vi "ParamReader2.vi"(8 "error in (no error)":errorcluster, 10 "what kind of binary":i32, 11 "selected path":path caption="selected \"*.par\" path") -> (0 "error out":errorcluster, 2 "CodeString":string, 5 "Cluster":T1 {"AdcOffset" format="%#.6f"; "AdcScale" format="%#.6f"})   [LabVIEW 2014]
panel:
  out "slow ADC\nactiveChannels\nRange":string
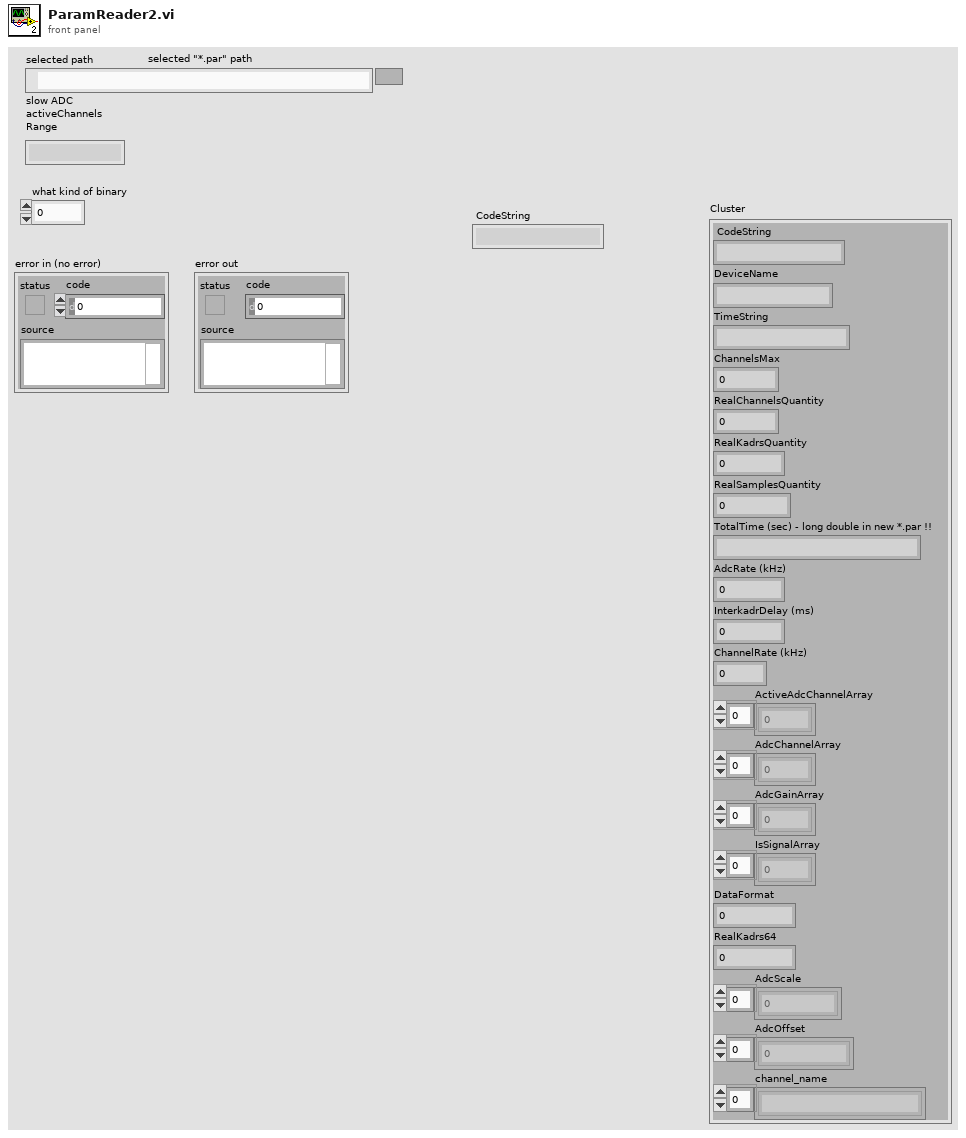
[diagram p1: front panel]
types:
  T1 = cluster{" CodeString":string, "DeviceName":string, "TimeString":string, "ChannelsMax":i16, "RealChannelsQuantity":i16, "RealKadrsQuantity":i64, "RealSamplesQuantity":i64, "TotalTime (sec) - long double in new *.par !!":string, "AdcRate (kHz)":dbl, "InterkadrDelay (ms)":dbl, "ChannelRate (kHz)":dbl, "ActiveAdcChannelArray":u32[], "AdcChannelArray":u8[], "AdcGainArray":u8[], "IsSignalArray":u8[], "DataFormat":i32, "RealKadrs64":i64, "AdcScale":dbl[], "AdcOffset":dbl[], "channel_name":string[]}
  T2 = enum16{"open", "replace", "create", "open or create", "replace or create", "replace or create with confirmation"}
  T3 = enum16{"deny read/write", "deny write-only", "deny none"}
  T4 = enum16{"big-endian, network order", "native, host order", "little-endian"}
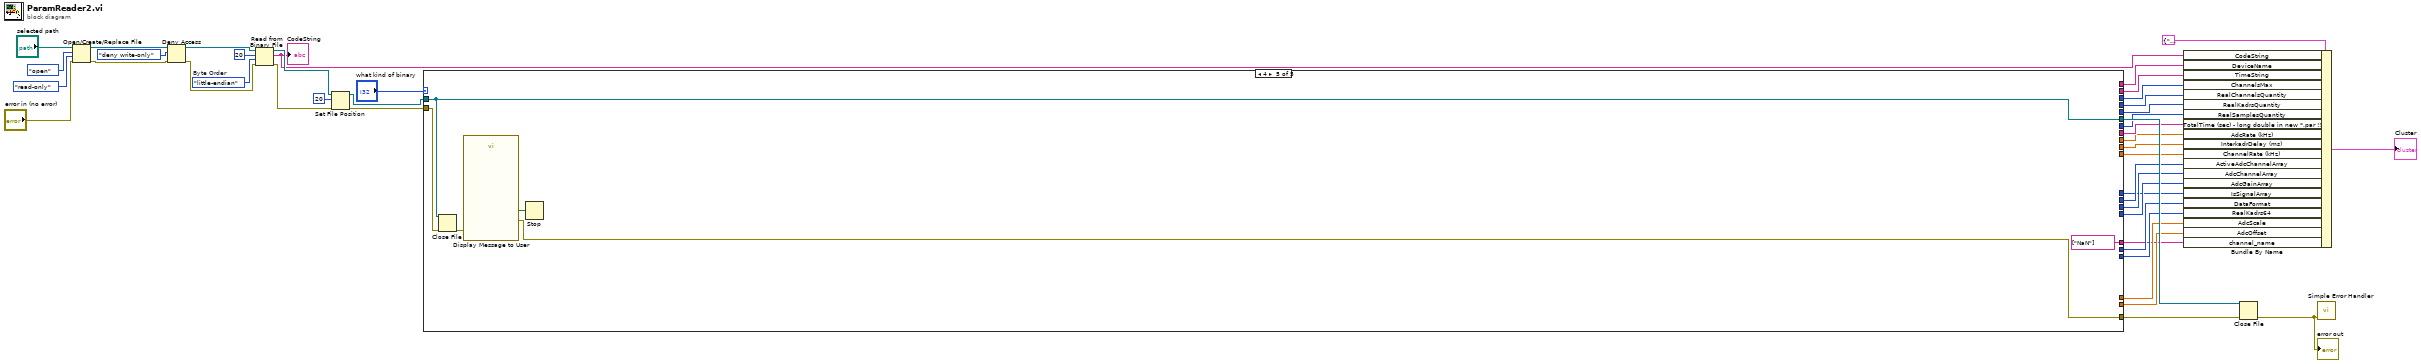
[diagram p0: block diagram]
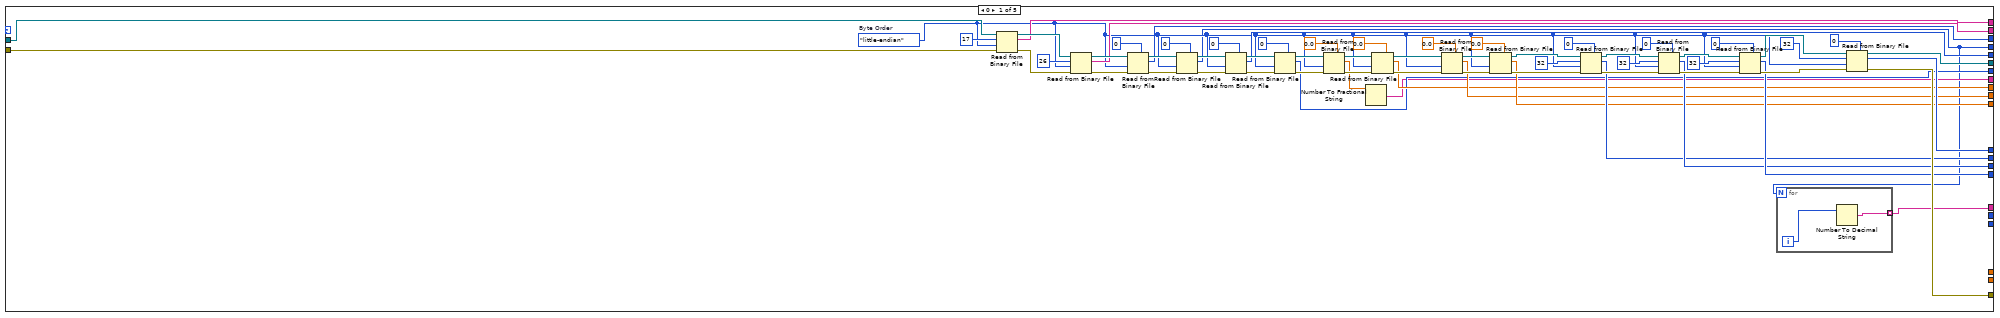
[diagram p2: hidden frame]
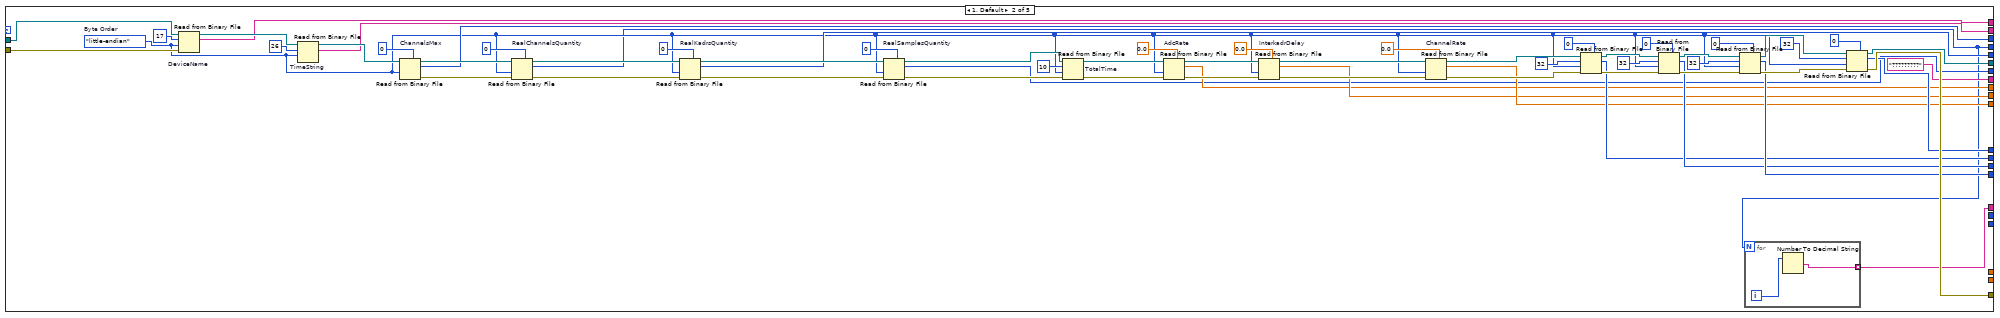
[diagram p3: hidden frame]
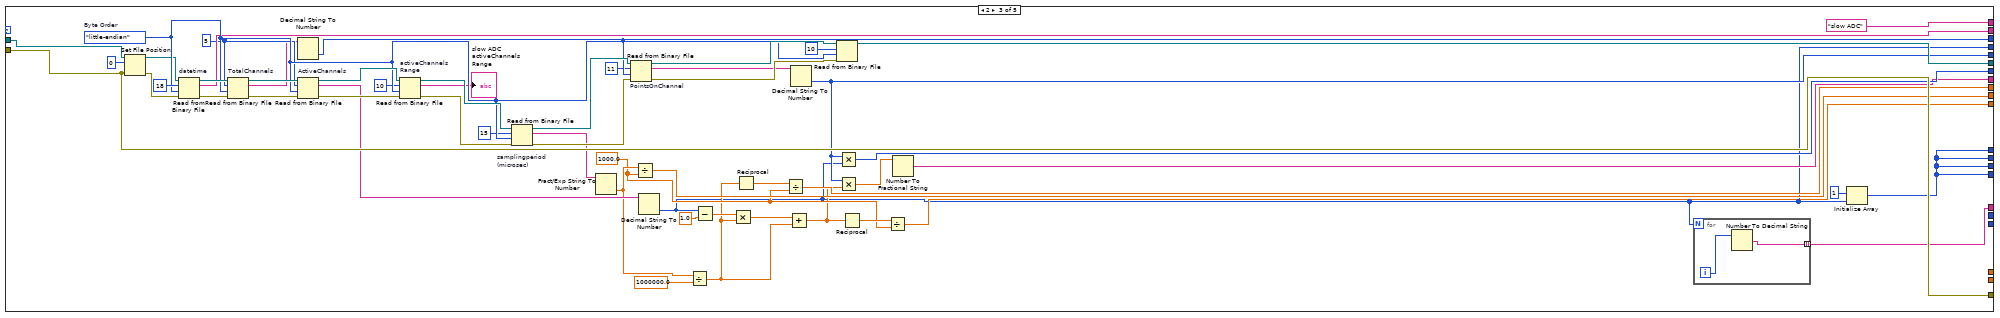
[diagram p4: hidden frame]
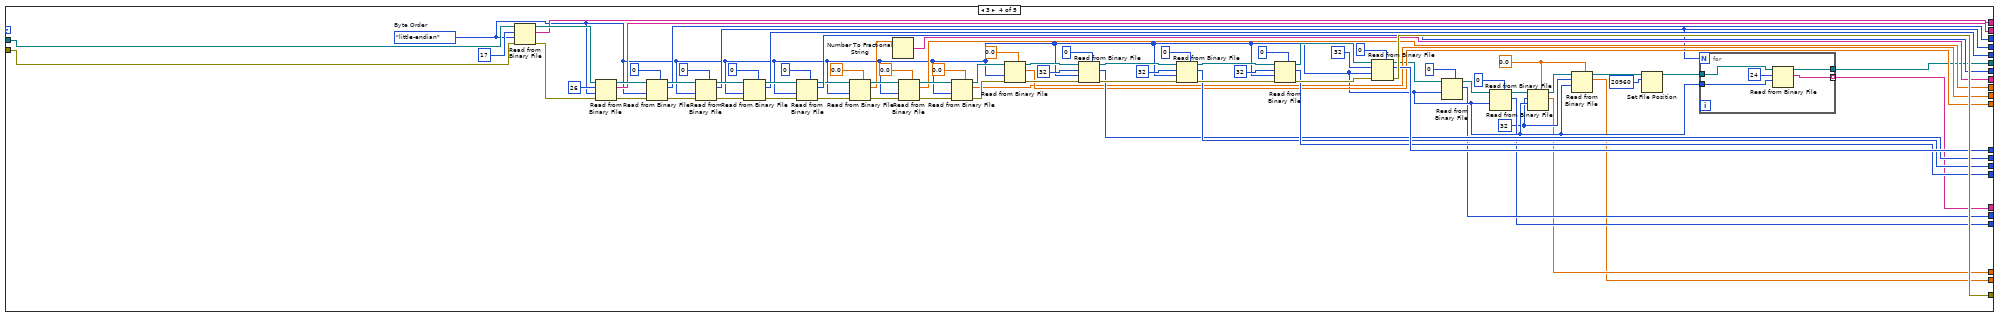
[diagram p5: hidden frame]
diagram:
  w29 = T4."little-endian"  # Byte Order
  n1 = Open/Create/Replace File(file path (use dialog)="selected path", error in="error in (no error)", operation (0:open)=T2."open", access (0:read/write)=enum16{"read/write", "read-only", "write-only"}."read-only") -> (refnum out=w31:refnum<file>, error out=w30:errorcluster)  [unwired: 2 in, 1 out]
  n2 = Deny Access(4:w30, 6:T3."deny write-only" ("deny mode (0:deny read/write)"), 7:w31) -> (0:w35:errorcluster, 3:w34:refnum<file>)
  n3 = Read from Binary File(8:w35, 9:w29, 10:20 ("count (1)"), 11:w34) -> (0:w39:errorcluster, 2:w20:string, 3:w37:refnum<file>)  [unwired: 2 in, 1 out]
  "CodeString" <- w20
  n4 = Set File Position(offset (in bytes) (0)=i64 20, refnum=w37, error in=w39) -> (refnum out=w41:refnum<file>, error out=w40:errorcluster)  [unwired: 1 in]
  n5 = case shown="4" "what kind of binary" {
    tunnel: w41 -> [w107 w171 w212 w309 w316]
    tunnel: [w66 w127 w208 w268 w318] -> w36
    tunnel: w40 -> [w106 w170 w208 w308 w320]
    tunnel: [w65 w126 w205 w248 w316] -> w42
    tunnel: [w64 w125 w185 w267 _] -> w6
    tunnel: [w63 w124 w185 w266 _] -> w7
    tunnel: [w62 w123 w185 w265 _] -> w8
    tunnel: [w61 w122 w185 w264 _] -> w9
    tunnel: [w60 w121 w181 w263 _] -> w10
    tunnel: [w59 w120 w189 w262 _] -> w11
    tunnel: [w58 w119 w191 w261 _] -> w12
    tunnel: [w57 w118 w190 w260 _] -> w14
    tunnel: [w56 w117 w177 w259 _] -> w15
    tunnel: [w44 w110 w174 w246 _] -> w16
    tunnel: [w55 w116 w198 w247 _] -> w17
    tunnel: [w54 w115 w207 w258 _] -> w18
    tunnel: [w53 w114 "slow ADC" w257 _] -> w19
    tunnel: [w49 "?????????" w178 w253 _] -> w13
    tunnel: [w43 w111 w175 w245 string[] ["NaN"]] -> w1
    tunnel: [_ _ _ w235 _] -> w5
    tunnel: [_ _ _ w234 _] -> w4
    tunnel: [_ _ _ w231 _] -> w3
    tunnel: [_ _ _ w230 _] -> w2
    frame 0 {
      w45 = T4."little-endian"  # Byte Order
      n6 = Read from Binary File(8:w106, 9:w45, 10:17 ("count (1)"), 11:w107) -> (0:w46:errorcluster, 2:w53:string, 3:w103:refnum<file>)  [unwired: 2 in, 1 out]
      n7 = Read from Binary File(8:w46, 9:w45, 10:26 ("count (1)"), 11:w103) -> (0:w47:errorcluster, 2:w54:string, 3:w101:refnum<file>)  [unwired: 2 in, 1 out]
      n8 = Read from Binary File(5:i16 0 ("count (1)"), 8:w47, 9:w45, 11:w101) -> (0:w88:errorcluster, 2:w55:i16, 3:w99:refnum<file>)  [unwired: 2 in, 1 out]
      n9 = Read from Binary File(5:i16 0 ("count (1)"), 8:w88, 9:w45, 11:w99) -> (0:w93:errorcluster, 2:w44:i16, 3:w92:refnum<file>)  [unwired: 2 in, 1 out]
      n10 = Read from Binary File(5:0 ("count (1)"), 8:w93, 9:w45, 11:w92) -> (0:w90:errorcluster, 2:w56:i32, 3:w91:refnum<file>)  [unwired: 2 in, 1 out]
      n11 = Read from Binary File(5:0 ("count (1)"), 8:w90, 9:w45, 11:w91) -> (0:w89:errorcluster, 2:w57:i32, 3:w51:refnum<file>)  [unwired: 2 in, 1 out]
      n12 = Read from Binary File(5:0.0 ("count (1)"), 8:w89, 9:w45, 11:w51) -> (0:w85:errorcluster, 2:w48:dbl, 3:w50:refnum<file>)  [unwired: 2 in, 1 out]
      n13 = Number To Fractional String(number=w48) -> (F-format string=w49:string)  [unwired: 3 in]
      n14 = Read from Binary File(5:sgl 0.0 ("count (1)"), 8:w85, 9:w45, 11:w50) -> (0:w84:errorcluster, 2:w58:sgl, 3:w87:refnum<file>)  [unwired: 2 in, 1 out]
      n15 = Read from Binary File(5:sgl 0.0 ("count (1)"), 8:w84, 9:w45, 11:w87) -> (0:w83:errorcluster, 2:w59:sgl, 3:w86:refnum<file>)  [unwired: 2 in, 1 out]
      n16 = Read from Binary File(5:sgl 0.0 ("count (1)"), 8:w83, 9:w45, 11:w86) -> (0:w79:errorcluster, 2:w60:sgl, 3:w80:refnum<file>)  [unwired: 2 in, 1 out]
      n17 = Read from Binary File(5:u8 0 ("count (1)"), 8:w79, 9:w45, 10:32 ("count (1)"), 11:w80) -> (0:w69:errorcluster, 2:w61:u8[], 3:w72:refnum<file>)  [unwired: 1 in, 1 out]
      n18 = Read from Binary File(5:u8 0 ("count (1)"), 8:w69, 9:w45, 10:32 ("count (1)"), 11:w72) -> (0:w68:errorcluster, 2:w62:u8[], 3:w71:refnum<file>)  [unwired: 1 in, 1 out]
      n19 = Read from Binary File(5:u8 0 ("count (1)"), 8:w68, 9:w45, 10:32 ("count (1)"), 11:w71) -> (0:w67:errorcluster, 2:w63:u8[], 3:w70:refnum<file>)  [unwired: 1 in, 1 out]
      n20 = for {
        N: w44 -> [_]
        tunnel: [w109] -> w43 mode=indexing
        i -> [w108]
        n21 = Number To Decimal String(number=w108) -> (decimal integer string=w109:string)  [unwired: 1 in]
      }
      n22 = Read from Binary File(5:u8 0 ("count (1)"), 8:w67, 9:w45, 10:32 ("count (1)"), 11:w70) -> (0:w66:errorcluster, 2:w64:u8[], 3:w65:refnum<file>)  [unwired: 1 in, 1 out]
    }
    frame 1, Default {
      w112 = T4."little-endian"  # Byte Order
      n23 = Read from Binary File "DeviceName"(8:w170, 9:w112, 10:17 ("count (1)"), 11:w171) -> (2:w114:string, 3:w167:refnum<file>)  [unwired: 2 in, 2 out]
      n24 = Read from Binary File "TimeString"(9:w112, 10:26 ("count (1)"), 11:w167) -> (2:w115:string, 3:w165:refnum<file>)  [unwired: 3 in, 2 out]
      n25 = Read from Binary File "ChannelsMax"(5:i16 0 ("count (1)"), 9:w112, 11:w165) -> (0:w150:errorcluster, 2:w116:i16, 3:w163:refnum<file>)  [unwired: 3 in, 1 out]
      n26 = Read from Binary File "RealChannelsQuantity"(5:i16 0 ("count (1)"), 8:w150, 9:w112, 11:w163) -> (0:w156:errorcluster, 2:w110:i16, 3:w155:refnum<file>)  [unwired: 2 in, 1 out]
      n27 = Read from Binary File "RealKadrsQuantity"(5:i64 0 ("count (1)"), 8:w156, 9:w112, 11:w155) -> (0:w152:errorcluster, 2:w117:i64, 3:w154:refnum<file>)  [unwired: 2 in, 1 out]
      n28 = Read from Binary File "RealSamplesQuantity"(5:i64 0 ("count (1)"), 8:w152, 9:w112, 11:w154) -> (0:w151:errorcluster, 2:w118:i64, 3:w153:refnum<file>)  [unwired: 2 in, 1 out]
      n29 = Read from Binary File "TotalTime"(8:w151, 9:w112, 10:10 ("count (1)"), 11:w153) -> (0:w146:errorcluster, 3:w149:refnum<file>)  [unwired: 2 in, 2 out]
      n30 = Read from Binary File "AdcRate"(5:0.0 ("count (1)"), 8:w146, 9:w112, 11:w149) -> (0:w145:errorcluster, 2:w119:dbl, 3:w148:refnum<file>)  [unwired: 2 in, 1 out]
      n31 = Read from Binary File "InterkadrDelay"(5:0.0 ("count (1)"), 8:w145, 9:w112, 11:w148) -> (0:w144:errorcluster, 2:w120:dbl, 3:w147:refnum<file>)  [unwired: 2 in, 1 out]
      n32 = Read from Binary File "ChannelRate"(5:0.0 ("count (1)"), 8:w144, 9:w112, 11:w147) -> (0:w140:errorcluster, 2:w121:dbl, 3:w141:refnum<file>)  [unwired: 2 in, 1 out]
      n33 = Read from Binary File(5:u32 0 ("count (1)"), 8:w140, 9:w112, 10:32 ("count (1)"), 11:w141) -> (0:w130:errorcluster, 2:w122:u32[], 3:w133:refnum<file>)  [unwired: 1 in, 1 out]
      n34 = Read from Binary File(5:u8 0 ("count (1)"), 8:w130, 9:w112, 10:32 ("count (1)"), 11:w133) -> (0:w129:errorcluster, 2:w123:u8[], 3:w132:refnum<file>)  [unwired: 1 in, 1 out]
      n35 = Read from Binary File(5:u8 0 ("count (1)"), 8:w129, 9:w112, 10:32 ("count (1)"), 11:w132) -> (0:w128:errorcluster, 2:w124:u8[], 3:w131:refnum<file>)  [unwired: 1 in, 1 out]
      n36 = for {
        N: w110 -> [_]
        tunnel: [w173] -> w111 mode=indexing
        i -> [w172]
        n37 = Number To Decimal String(number=w172) -> (decimal integer string=w173:string)  [unwired: 1 in]
      }
      n38 = Read from Binary File(5:u8 0 ("count (1)"), 8:w128, 9:w112, 10:32 ("count (1)"), 11:w131) -> (0:w127:errorcluster, 2:w125:u8[], 3:w126:refnum<file>)  [unwired: 1 in, 1 out]
    }
    frame 2 {
      w187 = 1000.0 ("y")
      w204 = 5 ("count (1)")
      w215 = T4."little-endian"  # Byte Order
      n39 = Set File Position(offset (in bytes) (0)=i64 0, refnum=w212, error in=w208) -> (refnum out=w210:refnum<file>, error out=w209:errorcluster)  [unwired: 1 in]
      n40 = Read from Binary File "datetime"(8:w209, 9:w215, 10:18 ("count (1)"), 11:w210) -> (0:w214:errorcluster, 2:w207:string, 3:w226:refnum<file>)  [unwired: 2 in, 1 out]
      n41 = Read from Binary File "TotalChannels"(8:w214, 9:w215, 10:w204, 11:w226) -> (0:w213:errorcluster, 2:w200:string, 3:w225:refnum<file>)  [unwired: 2 in, 1 out]
      n42 = Decimal String To Number(string=w200) -> (number=w198:i32)  [unwired: 2 in, 1 out]
      n43 = Read from Binary File "ActiveChannels"(8:w213, 9:w215, 10:w204, 11:w225) -> (0:w216:errorcluster, 2:w199:string, 3:w224:refnum<file>)  [unwired: 2 in, 1 out]
      n44 = Read from Binary File "activeChannels\nRange"(8:w216, 9:w215, 10:10 ("count (1)"), 11:w224) -> (0:w222:errorcluster, 2:→"slow ADC\nactiveChannels\nRange":string, 3:w221:refnum<file>)  [unwired: 2 in, 1 out]
      n45 = Read from Binary File "samplingperiod\n(microsec)"(8:w222, 9:w215, 10:i64 15 ("count (1)"), 11:w221) -> (0:w218:errorcluster, 2:w195:string, 3:w220:refnum<file>)  [unwired: 2 in, 1 out]
      n46 = Fract/Exp String To Number(string=w195) -> (number=w188:dbl)  [unwired: 3 in, 1 out]
      n47 = Read from Binary File "PointsOnChannel"(8:w218, 9:w215, 10:i64 11 ("count (1)"), 11:w220) -> (0:w217:errorcluster, 2:w197:string, 3:w219:refnum<file>)  [unwired: 2 in, 1 out]
      n48 = Divide(x=w188, y=w187) -> (x/y=w189:dbl)
      n49 = Decimal String To Number(string=w199) -> (number=w174:i32)  [unwired: 2 in, 1 out]
      n50 = Divide(x=w188, y=1000000.0) -> (x/y=w180:dbl)
      n51 = Subtract(x=w174, y=1.0) -> (x-y=w183:dbl)
      n52 = Multiply(x=w183, y=w180) -> (x*y=w182:dbl)
      n53 = Reciprocal(x=w180) -> (1/x=w192:dbl)
      n54 = Divide(x=w192, y=w187) -> (x/y=w191:dbl)
      n55 = Add(x=w182, y=w180) -> (x+y=w176:dbl)
      n56 = Decimal String To Number(string=w197) -> (number=w177:i32)  [unwired: 2 in, 1 out]
      n57 = Read from Binary File(8:w217, 9:w215, 10:10 ("count (1)"), 11:w219) -> (3:w205:refnum<file>)  [unwired: 2 in, 3 out]
      n58 = Multiply(x=w177, y=w174) -> (x*y=w190:i32)
      n59 = Multiply(x=w177, y=w176) -> (x*y=w179:dbl)
      n60 = Reciprocal(x=w176) -> (1/x=w194:dbl)
      n61 = Divide(x=w194, y=w187) -> (x/y=w181:dbl)
      n62 = Number To Fractional String(number=w179) -> (F-format string=w178:string)  [unwired: 3 in]
      n63 = for {
        N: w174 -> [_]
        tunnel: [w229] -> w175 mode=indexing
        i -> [w228]
        n64 = Number To Decimal String(number=w228) -> (decimal integer string=w229:string)  [unwired: 1 in]
      }
      n65 = Initialize Array(i8 1 ("element"), w174) -> (w185:i8[])
    }
    frame 3 {
      w232 = 32 ("count (1)")
      w233 = 0.0 ("count (1)")
      w238 = T4."little-endian"  # Byte Order
      n66 = Read from Binary File(8:w308, 9:w238, 10:17 ("count (1)"), 11:w309) -> (0:w250:errorcluster, 2:w257:string, 3:w305:refnum<file>)  [unwired: 2 in, 1 out]
      n67 = Read from Binary File(8:w250, 9:w238, 10:26 ("count (1)"), 11:w305) -> (0:w251:errorcluster, 2:w258:string, 3:w303:refnum<file>)  [unwired: 2 in, 1 out]
      n68 = Read from Binary File(5:i16 0 ("count (1)"), 8:w251, 9:w238, 11:w303) -> (0:w290:errorcluster, 2:w247:i16, 3:w301:refnum<file>)  [unwired: 2 in, 1 out]
      n69 = Read from Binary File(5:i16 0 ("count (1)"), 8:w290, 9:w238, 11:w301) -> (0:w295:errorcluster, 2:w246:i16, 3:w294:refnum<file>)  [unwired: 2 in, 1 out]
      n70 = Read from Binary File(5:0 ("count (1)"), 8:w295, 9:w238, 11:w294) -> (0:w292:errorcluster, 2:w259:i32, 3:w293:refnum<file>)  [unwired: 2 in, 1 out]
      n71 = Read from Binary File(5:0 ("count (1)"), 8:w292, 9:w238, 11:w293) -> (0:w291:errorcluster, 2:w260:i32, 3:w255:refnum<file>)  [unwired: 2 in, 1 out]
      n72 = Read from Binary File(5:0.0 ("count (1)"), 8:w291, 9:w238, 11:w255) -> (0:w287:errorcluster, 2:w252:dbl, 3:w254:refnum<file>)  [unwired: 2 in, 1 out]
      n73 = Number To Fractional String(number=w252) -> (F-format string=w253:string)  [unwired: 3 in]
      n74 = Read from Binary File(5:sgl 0.0 ("count (1)"), 8:w287, 9:w238, 11:w254) -> (0:w286:errorcluster, 2:w261:sgl, 3:w289:refnum<file>)  [unwired: 2 in, 1 out]
      n75 = Read from Binary File(5:sgl 0.0 ("count (1)"), 8:w286, 9:w238, 11:w289) -> (0:w285:errorcluster, 2:w262:sgl, 3:w288:refnum<file>)  [unwired: 2 in, 1 out]
      n76 = Read from Binary File(5:sgl 0.0 ("count (1)"), 8:w285, 9:w238, 11:w288) -> (0:w281:errorcluster, 2:w263:sgl, 3:w282:refnum<file>)  [unwired: 2 in, 1 out]
      n77 = Read from Binary File(5:u8 0 ("count (1)"), 8:w281, 9:w238, 10:32 ("count (1)"), 11:w282) -> (0:w271:errorcluster, 2:w264:u8[], 3:w274:refnum<file>)  [unwired: 1 in, 1 out]
      n78 = Read from Binary File(5:u8 0 ("count (1)"), 8:w271, 9:w238, 10:32 ("count (1)"), 11:w274) -> (0:w270:errorcluster, 2:w265:u8[], 3:w273:refnum<file>)  [unwired: 1 in, 1 out]
      n79 = Read from Binary File(5:u8 0 ("count (1)"), 8:w270, 9:w238, 10:32 ("count (1)"), 11:w273) -> (0:w269:errorcluster, 2:w266:u8[], 3:w272:refnum<file>)  [unwired: 1 in, 1 out]
      n80 = Read from Binary File(5:u8 0 ("count (1)"), 8:w269, 9:w238, 10:32 ("count (1)"), 11:w272) -> (0:w268:errorcluster, 2:w267:u8[], 3:w243:refnum<file>)  [unwired: 1 in, 1 out]
      n81 = Read from Binary File(5:0 ("count (1)"), 9:w238, 11:w243) -> (2:w235:i32, 3:w242:refnum<file>)  [unwired: 3 in, 2 out]
      n82 = Read from Binary File(5:i64 0 ("count (1)"), 9:w238, 11:w242) -> (2:w234:i64, 3:w241:refnum<file>)  [unwired: 3 in, 2 out]
      n83 = Read from Binary File(5:w233, 9:w238, 10:w232, 11:w241) -> (2:w231:dbl[], 3:w240:refnum<file>)  [unwired: 2 in, 2 out]
      n84 = Read from Binary File(5:w233, 9:w238, 10:w232, 11:w240) -> (2:w230:dbl[], 3:w239:refnum<file>)  [unwired: 2 in, 2 out]
      n85 = Set File Position(offset (in bytes) (0)=i64 20960, refnum=w239) -> (refnum out=w244:refnum<file>)  [unwired: 2 in, 1 out]
      n86 = for {
        N: w246 -> [_]
        tunnel: w238 -> [w312]
        tunnel: w244 -> [w314]
        tunnel: [w313] -> w248
        tunnel: [w311] -> w245 mode=indexing
        n87 = Read from Binary File(9:w312, 10:24 ("count (1)"), 11:w314) -> (2:w311:string, 3:w313:refnum<file>)  [unwired: 3 in, 2 out]
      }
    }
    frame 4 {
      n88 = Close File(refnum=w316, error in=w320) -> (error out=w319:errorcluster)  [unwired: 1 out]
      n89 = call "Display Message to User"("error in (no error)"=w319) -> ("error out"=w318:errorcluster, "OK"=w317:bool)  [unwired: 9 in]
      n90 = Stop(stop? (T)=w317) -> ()
    }
  }
  n91 = Bundle By Name(cluster=T1 {" CodeString"="3571090,7859525  \u0000\u0000\u0000", "DeviceName"="E2010\u0000\u0000\u0000\u0000\u0000\u0000\u0000\u0000\u0000\u0000\u0000\u0000", "TimeString"="  02-10-2015 15:50:30\u0000\u0000\u0000\u0000\u0000", "ChannelsMax"=4, "RealChannelsQuantity"=4, "RealKadrsQuantity"=200000, "RealSamplesQuantity"=800000, "TotalTime (sec) - long double in new *.par !!"="0.080000", "AdcRate (kHz)"=2500.0, "InterkadrDelay (ms)"=9.999999747378752e-05, "ChannelRate (kHz)"=2500.0, "ActiveAdcChannelArray"=[1, 1, 1, 1, 0, 0, 0, 0, 0, 0, 0, 0, 0, 0, 0, 0, 0, 0, 0, 0, 0, 0, 0, 0, 0, 0, 0, 0, 0, 0, 0, 0], "AdcChannelArray"=[0, 1, 2, 3, 4, 5, 6, 7, 8, 9, 10, 11, 12, 13, 14, 15, 16, 17, 18, 19, 20, 21, 22, 23, 24, 25, 26, 27, 28, 29, 30, 31], "AdcGainArray"=[0, 0, 0, 0, 0, 0, 0, 0, 0, 0, 0, 0, 0, 0, 0, 0, 0, 0, 0, 0, 0, 0, 0, 0, 0, 0, 0, 0, 0, 0, 0, 0], "IsSignalArray"=[0, 0, 0, 0, 0, 0, 0, 0, 0, 0, 0, 0, 0, 0, 0, 0, 0, 0, 0, 0, 0, 0, 0, 0, 0, 0, 0, 0, 0, 0, 0, 0], "DataFormat"=3, "RealKadrs64"=200000, "AdcScale"=[1.1072238683700562, 1.1072763204574585, 1.107199788093567, 1.1072269678115845, 1.0556581020355225, 1.0552871227264404, 1.055243730545044, 1.0555833578109741, 1.0995646715164185, 1.0995484590530396, 1.0996085405349731, 1.099328875541687, 1.0, 1.0, 1.0, 1.0, 1.0, 1.0, 1.0, 1.0, 1.0, 1.0, 1.0, 1.0, 1.0, 1.0, 1.0, 1.0, 1.0, 1.0, 1.0, 1.0], "AdcOffset"=[-8.893548965454102, -8.418173789978027, -7.680645942687988, -9.022905349731445, -1.0585507154464722, 1.6397662162780762, 1.4740158319473267, -0.589760959148407, 81.70808410644531, 95.51783752441406, 84.60665893554688, 83.73567962646484, 0.0, 0.0, 0.0, 0.0, 0.0, 0.0, 0.0, 0.0, 0.0, 0.0, 0.0, 0.0, 0.0, 0.0, 0.0, 0.0, 0.0, 0.0, 0.0, 0.0], "channel_name"=["", "", "", "", "", "", "", "", "", "", "", "", "", "", "", "", "", "", "", "", "", "", "", "", "", "", "", "", "", "", "", "", "0"]} ("Cluster 2"), "CodeString"=w20, "DeviceName"=w19, "TimeString"=w18, "ChannelsMax"=w17, "RealChannelsQuantity"=w16, "RealKadrsQuantity"=w15, "RealSamplesQuantity"=w14, "TotalTime (sec) - long double in new *.par !!"=w13, "AdcRate (kHz)"=w12, "InterkadrDelay (ms)"=w11, "ChannelRate (kHz)"=w10, "ActiveAdcChannelArray"=w9, "AdcChannelArray"=w8, "AdcGainArray"=w7, "IsSignalArray"=w6, "DataFormat"=w5, "RealKadrs64"=w4, "AdcScale"=w3, "AdcOffset"=w2, "channel_name"=w1) -> (→"Cluster":T1)
  n92 = Close File(refnum=w42, error in=w36) -> (error out=w27:errorcluster)  [unwired: 1 out]
  "error out" <- w27
  n93 = call <vilib>:"Simple Error Handler.vi"("error in (no error)"=w27) -> ()  [unwired: 4 in, 5 out]
